vi "Remove.vi"(8 "error in (no error)":errorcluster, 9 "uService ID":string, 10 "Guardian":string, 11 "Distr uS Map ref in":refnum<data-value>) -> (0 "error out":errorcluster, 2 "List unchanged?":bool, 3 "Distr uS Map ref out":refnum<data-value>)   [LabVIEW 2026, in "TALOS.lvlib" / "Classes.lvlib" / "Distributed uService Map.lvclass"]
uses:
  Distributed uService Map.lvclass
  Distributed uService Map.lvclass/Distributed uService Map.ctl
  Ancestor/Ancestor/Ancestor.lvclass/Ancestor.ctl
  Support VIs/Generate Error.vi
  FGV/Error Memory/Get Error Description.vi
  Support VIs/Get PC name.vi
  Ancestor/Ancestor/Read ID.vi
  Support VIs/Get Class Name.vi
  <vilib>/Utility/error.llb/Clear Errors.vi
  FGV/Error Memory/Error Memory Core.vi
  <vilib>/AdvancedString/Delimited String to 1D String Array.vi
  <vilib>/AdvancedString/Delimited String to 1D String Array (string).vi
  Support VIs/Circus Root Path.vi
  FGV/Error Memory/Error Crt Lvl checker.vi
  FGV/Error Memory/Error Memory Core.vi/40c8088d-b597-4017-91af-faa98e00292e.vi
  FGV/Error Memory/Error Memory Core.vi/d4a3ab98-063c-4e44-b43d-fbdcfe6c2be2.vi
  Support VIs/Global Memory.vi
  <vilib>/Utility/LVClass/Get LV Class Name.vi
  Support VIs/Is in Packed Library.vi
  Support VIs/TALOS Root path.vi
  Support VIs/Read CSV worksheet.vi
  Support VIs/Global Constants.vi
  <vilib>/Utility/error.llb/General Error Handler.vi
  Support VIs/Error Log.vi
  Ancestor/Ancestor/Ancestor.lvclass
  <vilib>/Comparison/Equal/Equal Functor/Equal Functor.lvclass
  TALOS.lvlib
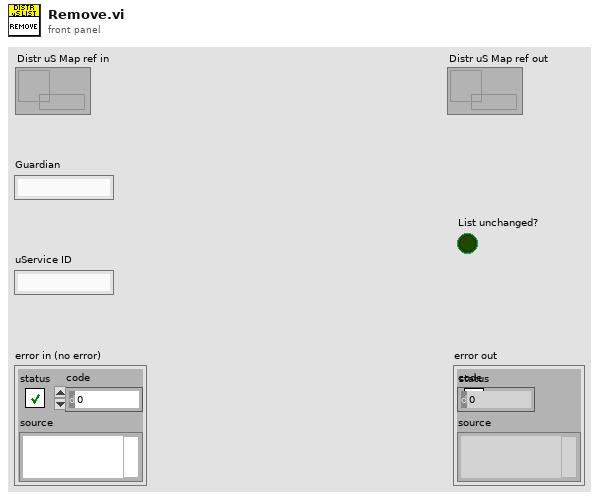
[diagram p1: front panel]
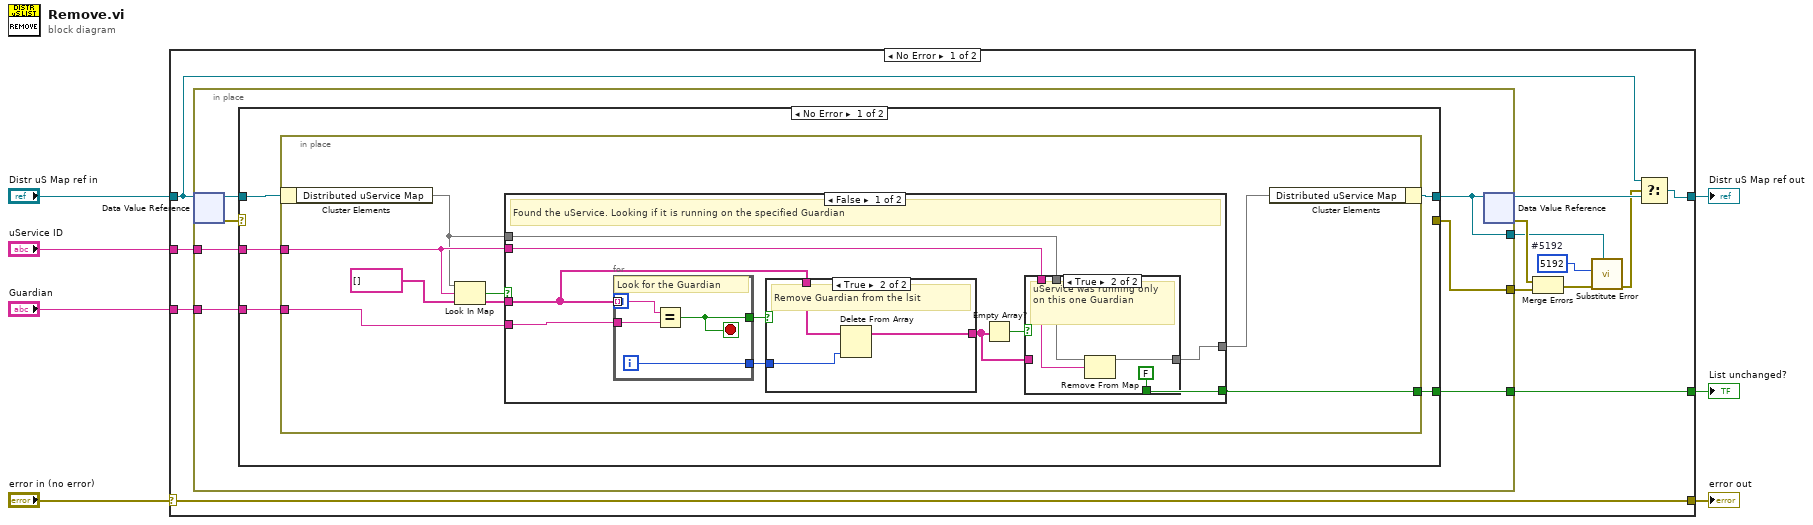
[diagram p0: block diagram]
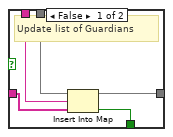
[diagram p2: hidden frame]
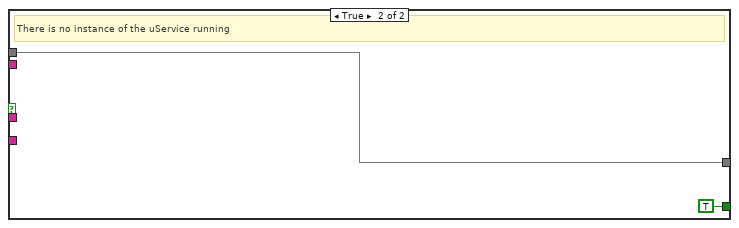
[diagram p4: hidden frame]
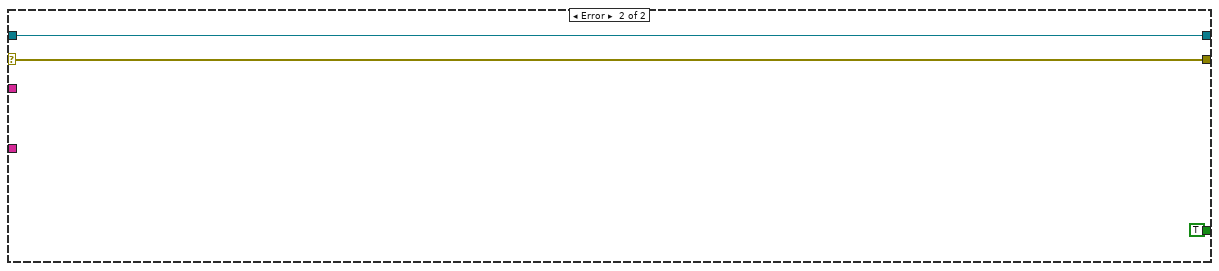
[diagram p5: hidden frame]
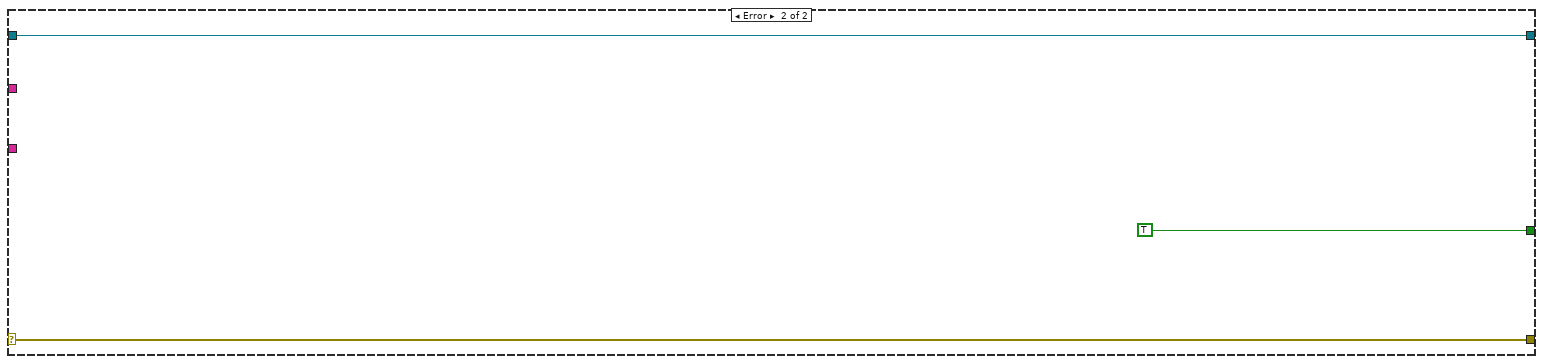
[diagram p6: hidden frame]
diagram:
  n1 = case shown="No Error" "error in (no error)" {
    selector: "error in (no error)" -> [w20 w75]
    tunnel: [w20 w75] -> w6
    tunnel: [w10 w74] -> w2
    tunnel: "Distr uS Map ref in" -> [w8 w74]
    tunnel: "uService ID" -> [w18 _]
    tunnel: "Guardian" -> [w19 _]
    tunnel: [w17 TRUE ("value unchanged?")] -> w3
    frame No Error {
      w12 = 5192  # #5192
      n2 = in-place {
        in-place-border: w19 -> [w27]
        in-place-border: w18 -> [w26]
        in-place-border: [w25] -> w17
        in-place-border: [w22] -> w15
        in-place-border: [w21] -> w13
        n3 = in-place-dvr #1(w8) -> (w24:refnum<class "Distributed uService Map.lvclass">, w23:errorcluster)
        n4 = case shown="No Error" w23 {
          selector: w23 -> [_ w70]
          tunnel: w27 -> [w32 _]
          tunnel: w26 -> [w31 _]
          tunnel: [w30 TRUE ("value unchanged?")] -> w25
          tunnel: w24 -> [w29 w72]
          tunnel: [w28 w72] -> w21
          tunnel: [_ w70] -> w22
          frame No Error {
            n5 = in-place {
              in-place-border: w32 -> [w38]
              in-place-border: w31 -> [w37]
              in-place-border: [w35] -> w30
              n6 = in-place-cluster #2(w29) -> ("Distributed uService Map"=w34:map{string, string[]})
              n7 = Look In Map(map=w34, key=w37, default value=string[] []) -> (key not found?=w40:bool, value=w39:string[])
              n8 = case shown="False" w40 {
                tunnel: w39 -> [w48 _]
                tunnel: w38 -> [w49 _]
                tunnel: w37 -> [w44 _]
                tunnel: w34 -> [w45 w69]
                tunnel: [w43 w69] -> w33
                tunnel: [w41 TRUE ("value unchanged?")] -> w35
                frame False {
                  # "Found the uService. Looking if it is running on the specified Guardian"
                  n9 = for {
                    tunnel: w48 -> [w53] mode=indexing
                    tunnel: w49 -> [w54]
                    tunnel: [w51] -> w50
                    tunnel: [w52] -> w47
                    i -> [w52]
                    stop <- w51 stop-if-true
                    # "Look for the Guardian"
                    n10 = Equal?(x=w53, y=w54) -> (x = y?=w51:bool)
                  }
                  n11 = case shown="True" w50 {
                    tunnel: w48 -> [w64 w67]
                    tunnel: [w64 w65] -> w42
                    tunnel: w47 -> [_ w66]
                    frame False {
                      # "The uService is not runnig on the Guardian"
                    }
                    frame True {
                      # "Remove Guardian from the lsit"
                      n12 = Delete From Array(array=w67, index=w66) -> (array with subset deleted=w65:string[])  [unwired: 1 in, 1 out]
                    }
                  }
                  n13 = Empty Array?(array=w42) -> (empty?=w46:bool)
                  n14 = case shown="True" w46 {
                    tunnel: w45 -> [w59 w63]
                    tunnel: w44 -> [w58 w62]
                    tunnel: [w56 w61] -> w43
                    tunnel: w42 -> [w57 _]
                    tunnel: [w55 FALSE ("value unchanged?")] -> w41
                    frame False {
                      # "Update list of Guardians"
                      n15 = Insert Into Map(map in=w59, key=w58, value=w57) -> (map out=w56:map{string, string[]}, value unchanged?=w55:bool)  [unwired: 1 out]
                    }
                    frame True {
                      # "uService was running only on this one Guardian"
                      n16 = Remove From Map(10:w62, 11:w63) -> (3:w61:map{string, string[]})  [unwired: 2 out]
                    }
                  }
                }
                frame True {
                  # "There is no instance of the uService running"
                }
              }
              n17 = in-place-cluster #2("Distributed uService Map"=w33) -> (w28:refnum<class "Distributed uService Map.lvclass">)
            }
          }
          frame Error {
          }
        }
        n18 = in-place-dvr #1(w21) -> (w11:refnum<data-value>, w16:errorcluster)
      }
      n19 = Merge Errors(w16, w15) -> (w14:errorcluster)
      n20 = call "Substitute Error.vi"("LabVIEW Object"=w13, "error in (no error)"=w14, "Error Code"=w12) -> ("error out"=w9:errorcluster)  [unwired: 8 in]
      n21 = Select(t=w8, s=w9, f=w11) -> (s? t:f=w10:refnum<data-value>)
    }
    frame Error {
    }
  }
  "error out" <- w6
  "List unchanged?" <- w3
  "Distr uS Map ref out" <- w2
